vi "getImaginary.vi"(8 "error in (no error)":errorcluster, 11 "IComplexNumber in":refnum<class "IComplexNumber.lvclass">) -> (0 "error out":errorcluster, 2 "Complex Imaginary out":dbl, 3 "IComplexNumber out":refnum<class "IComplexNumber.lvclass">)   [LabVIEW 2022 SP3, in "openDAQ.lvlib" / "daqCoreTypes.lvlib" / "IComplexNumber.lvclass"]
uses:
  <instrlib>/openDAQ/Public/Classes/daqCoreTypes/IComplexNumber/IComplexNumber.lvclass
  C:/Program Files (x86)/National Instruments/LabVIEW 2022/instr.lib/openDAQ/Public/Classes/IBaseObject/IBaseObject.lvclass
  <instrlib>/openDAQ/Public/Classes/IBaseObject/IBaseObject.lvclass/IBaseObject.ctl
  <instrlib>/openDAQ/Public/Classes/IBaseObject/Accessor/Read reference.vi
  <instrlib>/openDAQ/Binaries/Windows/x86/copendaq32.dll
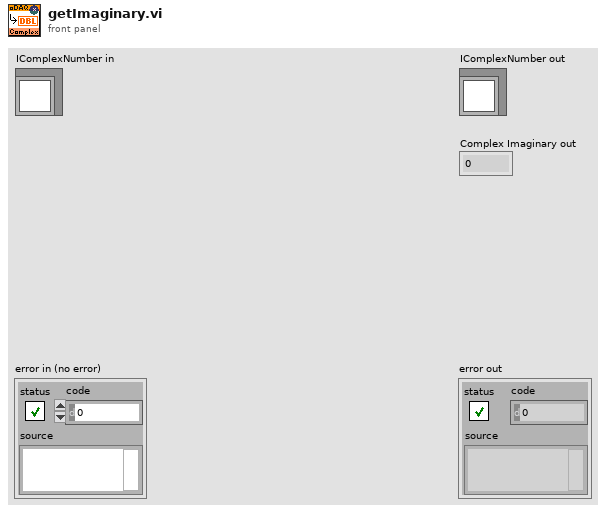
[diagram p1: front panel]
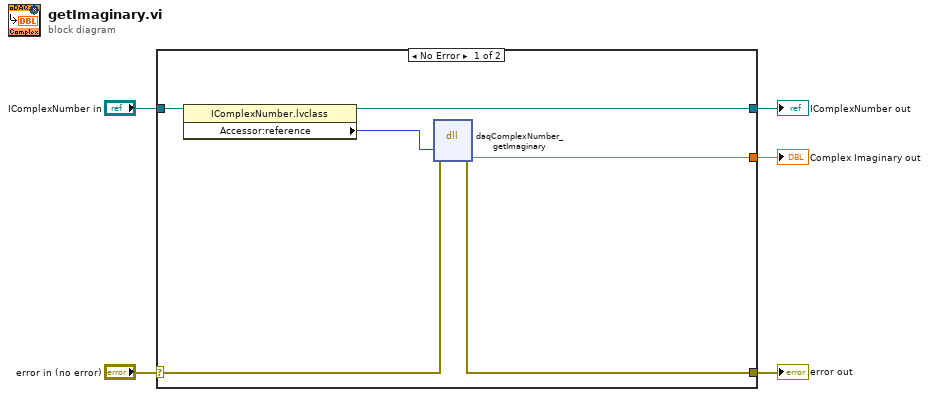
[diagram p0: block diagram]
diagram:
  n1 = case shown="No Error" "error in (no error)" {
    selector: "error in (no error)" -> [w10 w13]
    tunnel: [w9 w13] -> w4
    tunnel: [w8 w12] -> w2
    tunnel: "IComplexNumber in" -> [w11 w12]
    tunnel: [w6 _] -> w1
    frame No Error {
      n2 = property class="IComplexNumber.lvclass"(reference=w11) -> (reference out=w8:refnum<class "IComplexNumber.lvclass">, "Accessor:reference"=w7:i64)  [unwired: 1 in, 1 out]
      n3 = dll-call lib="C:/Program Files (x86)/National Instruments/LabVIEW 2022/instr.lib/openDAQ/Binaries/Windows/x86/copendaq*.*" fn="daqComplexNumber_getImaginary"(error in=w10, "complexNumber"=w7) -> (error out=w9:errorcluster, "imaginary"=w6:dbl)  [unwired: 5 in, 1 out]
    }
    frame Error {
    }
  }
  "error out" <- w4
  "IComplexNumber out" <- w2
  "Complex Imaginary out" <- w1
